vi "PID Calibrator main.vi"() -> ()   [LabVIEW 2021]
panel:
  out "body.detectedObjectList":cluster{"name":string, "confidence":dbl}[](array[cluster])
  out "error out 2":errorcluster
  in  "Send":bool
  in  "payload":T1={"instructionID"=23, "leftWheelDistance"=300.0, "leftWheelSpeed"=100.0, "rightWheelDistance"=300.0, "rightWheelSpeed"=100.0, "time"=5.0, "object"=""}
  in  "Direct Method":string(combo)
  out "Delta":dbl(graph)
  out "error out":errorcluster
  out "Speed":T2(graph)
  out "Numeric":i32
  out "remote port":u16
  out "remote address":string
  in  "stop":bool
  in  "port":u16=2323
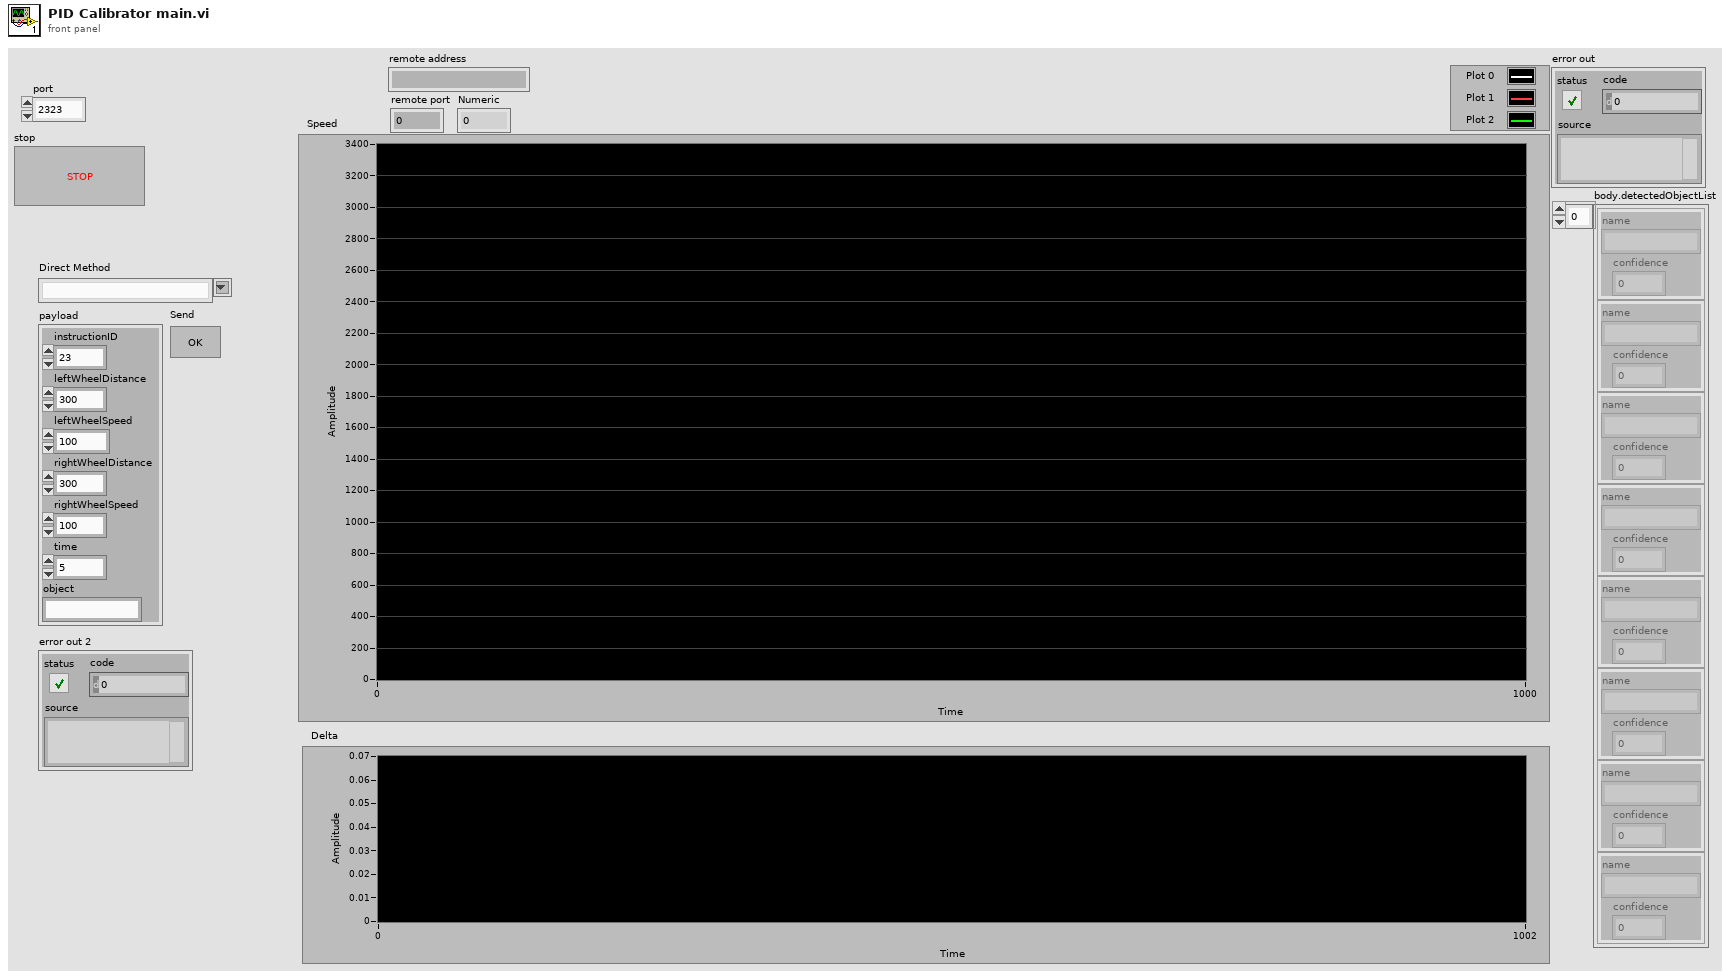
[diagram p1: front panel]
types:
  T1 = cluster{"instructionID":i32, "leftWheelDistance":dbl, "leftWheelSpeed":dbl, "rightWheelDistance":dbl, "rightWheelSpeed":dbl, "time":dbl, "object":string}
  T2 = cluster{"leftWheelSpeed":dbl, "rightWheelSpeed":dbl}
  T3 = enum16{"Standard", "Buffered", "CRLF", "Immediate"}
  T4 = cluster{"body":cluster{"leftWheelSpeed":dbl, "rightWheelSpeed":dbl, "sonarDistance":dbl, "detectedObjectList":cluster{"name":string, "confidence":dbl}[], "instructionID":i32}, "dataType":string, "deviceName":string}
  T5 = cluster{"method_name":string, "payload":cluster{"instructionID":i32, "leftWheelDistance":dbl, "leftWheelSpeed":dbl, "rightWheelDistance":dbl, "rightWheelSpeed":dbl, "time":dbl, "object":string}}
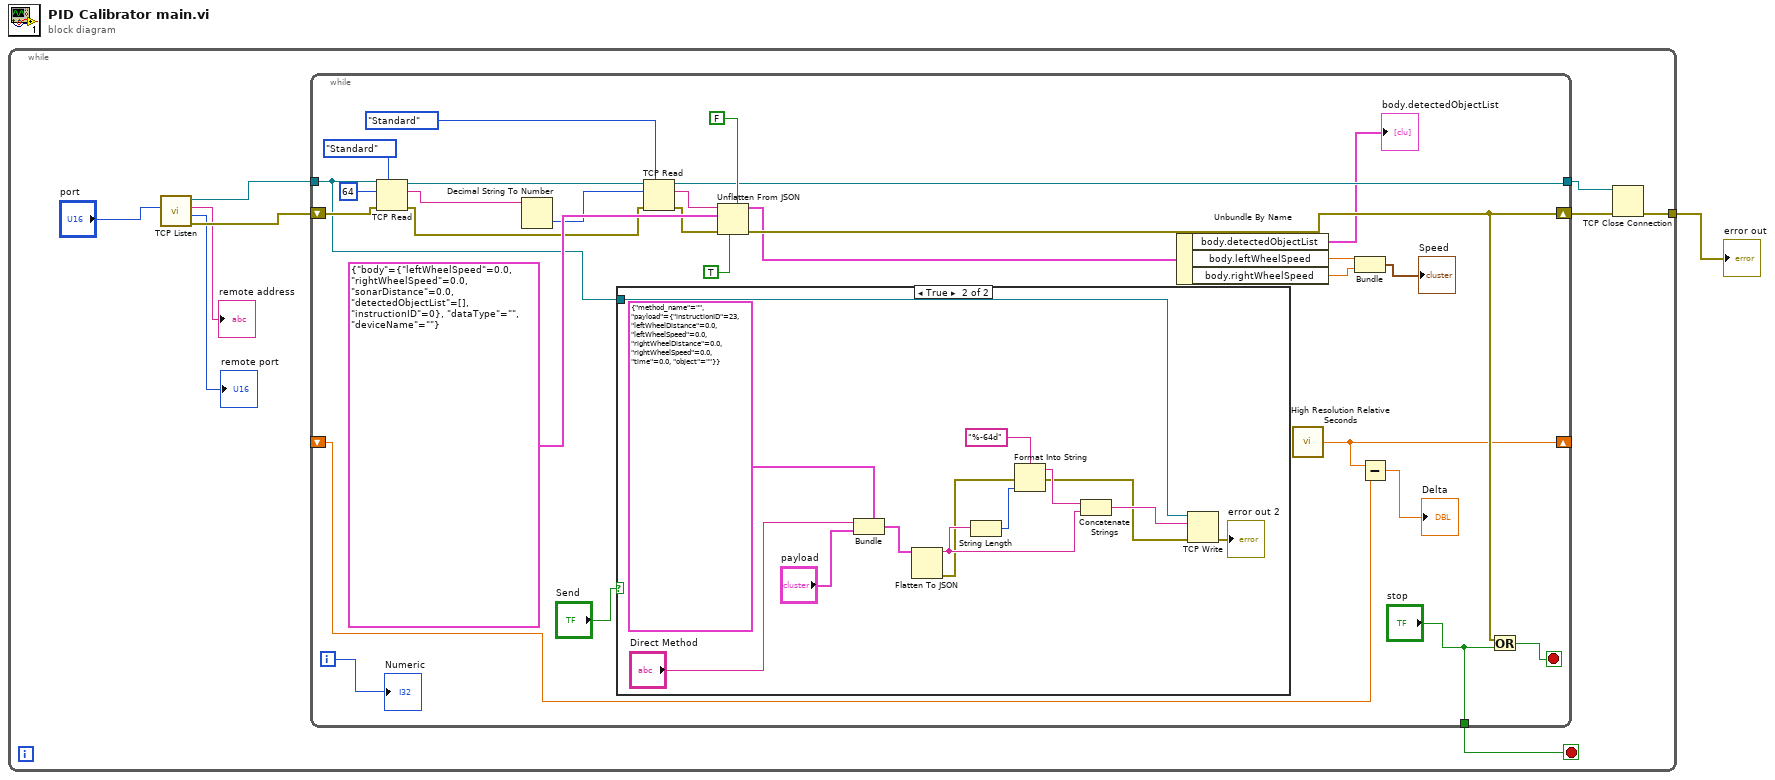
[diagram p0: block diagram]
diagram:
  n1 = while {
    tunnel: [w2] -> w1
    stop <- w3 stop-if-true
    n2 = call <vilib>:"TCP Listen.vi"("port"="port") -> ("error out"=w8:errorcluster, "remote port"=→"remote port":u16, "remote address"=→"remote address":string, "connection ID"=w9:refnum<k5>)  [unwired: 6 in, 1 out]
    n3 = while {
      tunnel: w9 -> [w12]
      tunnel: [w30] -> w7
      shift-right: [w23] -> w6
      shift-left: w8 -> [w25]
      tunnel: ["stop"] -> w3
      shift-right: [w14] -> _
      shift-left: _ -> [w16]
      i -> [w34]
      stop <- w24 stop-if-true
      n4 = TCP Read(connection ID=w12, bytes to read=64, error in (no error)=w25, 7:T3."Standard" ("mode (standard)")) -> (connection ID out=w33:refnum<k5>, data out=w29:string, error out=w27:errorcluster)  [unwired: 1 in]
      n5 = Decimal String To Number(string=w29) -> (number=w28:i32)  [unwired: 2 in, 1 out]
      n6 = case shown="True" "Send" {
        tunnel: w12 -> [_ w42]
        frame False {
        }
        frame True {
          n7 = Bundle(cluster=T5 {"method_name"="", "payload"={"instructionID"=23, "leftWheelDistance"=0.0, "leftWheelSpeed"=0.0, "rightWheelDistance"=0.0, "rightWheelSpeed"=0.0, "time"=0.0, "object"=""}}, "method_name"="Direct Method", "payload"="payload") -> (w48:T5)
          n8 = Flatten To JSON(anything=w48) -> (JSON string=w46:string, 11:w41:errorcluster)  [unwired: 2 in]
          n9 = String Length(string=w46) -> (length=w45:i32)
          n10 = Format Into String(format string="%-64d", error in=w41, w45) -> (resulting string=w47:string, error out=w40:errorcluster)  [unwired: 1 in]
          n11 = Concatenate Strings(w47, w46) -> (w43:string)
          n12 = TCP Write(connection ID=w42, data in=w43, error in (no error)=w40) -> (error out=→"error out 2":errorcluster)  [unwired: 1 in, 2 out]
        }
      }
      n13 = TCP Read(connection ID=w33, bytes to read=w28, error in (no error)=w27, 7:T3."Standard" ("mode (standard)")) -> (connection ID out=w30:refnum<k5>, data out=w31:string, error out=w26:errorcluster)  [unwired: 1 in]
      n14 = Unflatten From JSON(enable LabVIEW extensions? (T)=FALSE, JSON string=w31, type and defaults=T4 {"body"={"leftWheelSpeed"=0.0, "rightWheelSpeed"=0.0, "sonarDistance"=0.0, "detectedObjectList"=[], "instructionID"=0}, "dataType"="", "deviceName"=""}, default null elements? (F)=TRUE, error in (no error)=w26) -> (value=w20:T4, error out=w23:errorcluster)  [unwired: 2 in]
      n15 = Unbundle By Name(w20) -> ("body.detectedObjectList"=→"body.detectedObjectList":cluster{"name":string, "confidence":dbl}[], "body.leftWheelSpeed"=w19:dbl, "body.rightWheelSpeed"=w18:dbl)
      n16 = call <vilib>:"High Resolution Relative Seconds.vi"() -> ("relative seconds"=w14:dbl)
      n17 = Bundle("leftWheelSpeed"=w19, "rightWheelSpeed"=w18) -> (→"Speed":T2)  [unwired: 1 in]
      n18 = Subtract(x=w14, y=w16) -> (x-y=→"Delta":dbl)
      n19 = Or(x=w23, y="stop") -> (x .or. y?=w24:bool)
      "Numeric" <- w34
    }
    n20 = TCP Close Connection(connection ID=w7, error in (no error)=w6) -> (error out=w2:errorcluster)  [unwired: 1 in, 1 out]
  }
  "error out" <- w1
